vi "Enqueuer Control.vi"() -> ()   [LabVIEW 2020]
uses:
  Message Enqueuer/Message Enqueuer.lvclass
panel:
  in  "Enqueuer":refnum<class "Message Enqueuer.lvclass">
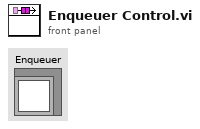
[diagram p1: front panel]
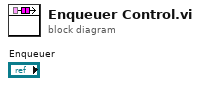
[diagram p0: block diagram]
diagram:
